vi "ep_Read Public Record Inf.vi"(8 "error in":errorcluster, 11 "task in":T2={"file refnums"=[], "Data Object"=refnum, "config info"={"station_name"="", "rec_dev_id"="", "rev_year"=1999.0, "TT"=0, "##A"=0, "##D"=0, "analog channel info"=[], "status channel info"=[], "lf"=50.0, "nrates"=0, "samp info"=[], "initial timestamp"=timestamp(0 s since 1904-01-01), "trigger timestamp"=timestamp(0 s since 1904-01-01), "ft"=enum."Binary", "timemult"=1.0}, "public inf content"={"Source"="", "Record Type"=enum."Unknown", "Phase ID"="", "Event Description"="", "Device ID"="", "Distance of Fault"=-1.0, "Distance Unit"=enum."Miles", "Max_Current"=inf, "Min_Current"=-inf, "Max_Voltage"=inf, "Min_Voltage"=-inf, "EventNoteCount"=0, "Event Information"=[]}, "private inf content"=[], "internal buffers"={"start index"=1, "config to public inf"=enum."disabled", "static config info"="", "static file_des record inf"="", "static file_des channel inf"="", "public inf"="", "private inf"=""}} {"public inf content"."Event Information"."min sample number" max=9999999999; "public inf content"."Event Information"."max sample number" max=9999999999; "config info"."nrates" max=999; "config info"."status channel info"."Dn" min=1 max=999999; "config info"."analog channel info"."An" min=1 max=999999; "config info"."trigger timestamp" format="%<%H:%M:%S%6u\n%d/%m/%Y>T"; "config info"."initial timestamp" format="%<%H:%M:%S%6u\n%d/%m/%Y>T"; "config info"."##D" max=999999; "config info"."##A" max=999999; "config info"."TT" min=1 max=999999; "config info"."rev_year" min=1999.0 max=1999.0}) -> (0 "error out":errorcluster, 2 "public record information":T1={"source"="", "record type"=enum."Unknown", "phase ID"="", "event description"="", "device ID"="", "distance of fault"=-1.0, "distance unit"=enum."Miles", "max current"=inf, "min current"=-inf, "max voltage"=inf, "min voltage"=-inf}, 3 "task out":T2={"file refnums"=[], "Data Object"=refnum, "config info"={"station_name"="", "rec_dev_id"="", "rev_year"=1999.0, "TT"=0, "##A"=0, "##D"=0, "analog channel info"=[], "status channel info"=[], "lf"=50.0, "nrates"=0, "samp info"=[], "initial timestamp"=timestamp(0 s since 1904-01-01), "trigger timestamp"=timestamp(0 s since 1904-01-01), "ft"=enum."Binary", "timemult"=1.0}, "public inf content"={"Source"="", "Record Type"=enum."Unknown", "Phase ID"="", "Event Description"="", "Device ID"="", "Distance of Fault"=-1.0, "Distance Unit"=enum."Miles", "Max_Current"=inf, "Min_Current"=-inf, "Max_Voltage"=inf, "Min_Voltage"=-inf, "EventNoteCount"=0, "Event Information"=[]}, "private inf content"=[], "internal buffers"={"start index"=1, "config to public inf"=enum."disabled", "static config info"="", "static file_des record inf"="", "static file_des channel inf"="", "public inf"="", "private inf"=""}} {"public inf content"."Event Information"."min sample number" max=9999999999; "public inf content"."Event Information"."max sample number" max=9999999999; "config info"."nrates" max=999; "config info"."status channel info"."Dn" min=1 max=999999; "config info"."analog channel info"."An" min=1 max=999999; "config info"."trigger timestamp" format="%<%H:%M:%S%6u\n%d/%m/%Y>T"; "config info"."initial timestamp" format="%<%H:%M:%S%6u\n%d/%m/%Y>T"; "config info"."##D" max=999999; "config info"."##A" max=999999; "config info"."TT" min=1 max=999999; "config info"."rev_year" min=1999.0 max=1999.0})   [LabVIEW 2011, in "NI_EP_COMTRADE.lvlib"]
uses:
  <vilib>/addons/Electrical Power/File IO/NI_EP_COMTRADE.lvlib
  <vilib>/addons/Electrical Power/File IO/COMTRADE/typedefs/ep_Task.ctl
  <vilib>/addons/Electrical Power/File IO/COMTRADE/typedefs/ep_Config Info.ctl
  <vilib>/addons/Electrical Power/File IO/COMTRADE/typedefs/ep_Analog Channel Info.ctl
  <vilib>/addons/Electrical Power/File IO/COMTRADE/typedefs/ep_Status Channel Info.ctl
  <vilib>/addons/Electrical Power/File IO/COMTRADE/typedefs/ep_File Format.ctl
  <vilib>/addons/Electrical Power/File IO/COMTRADE/typedefs/ep_Public Inf Content.ctl
  <vilib>/addons/Electrical Power/File IO/COMTRADE/typedefs/ep_Public Event Inf.ctl
  <vilib>/addons/Electrical Power/File IO/COMTRADE/typedefs/ep_Private Inf Content.ctl
  <vilib>/addons/Electrical Power/File IO/COMTRADE/typedefs/ep_Public Record Inf.ctl
  <vilib>/Platform/storage/Storage.llb/Get Property (Storage Refnums).vi
  <vilib>/Platform/storage/Storage.llb/Get Property (String).vi
  <vilib>/Platform/storage/Storage.llb/Get Property (DBL).vi
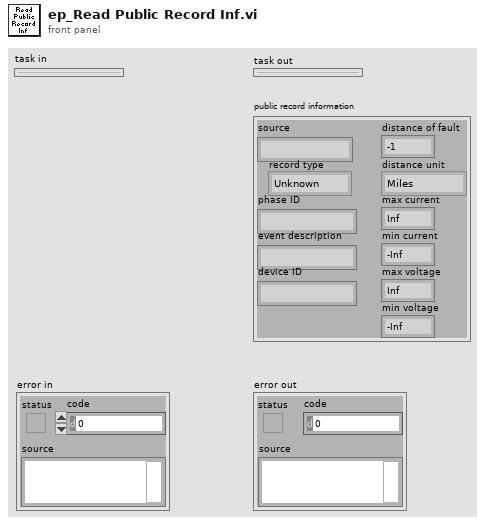
[diagram p1: front panel]
types:
  T1 = typedef "NI_EP_COMTRADE.lvlib/ep_Public Record Inf.ctl" = cluster{"source":string, "record type":enum16{"Fault", "Unknown", "Misoperation", "Close", "Trip", "Reclose", "Power swing", "Simulation"}, "phase ID":string, "event description":string, "device ID":string, "distance of fault":dbl, "distance unit":enum16{"Miles", "Kilometers", "Percent of line", "Percent of setting", "Ohms"}, "max current":dbl, "min current":dbl, "max voltage":dbl, "min voltage":dbl}
  T2 = typedef "NI_EP_COMTRADE.lvlib/ep_Task.ctl" = cluster{"file refnums":refnum<file>[], "Data Object":refnum<k20>, "config info":T3, "public inf content":T7, "private inf content":T9, "internal buffers":cluster{"start index":u32, "config to public inf":enum16{"disabled", "enabled", "buffered"}, "static config info":string, "static file_des record inf":string, "static file_des channel inf":string, "public inf":string, "private inf":string}}
  T3 = typedef "NI_EP_COMTRADE.lvlib/ep_Config Info.ctl" = cluster{"station_name":string, "rec_dev_id":string, "rev_year":dbl, "TT":u32, "##A":u32, "##D":u32, "analog channel info":T4[], "status channel info":T5[], "lf":sgl, "nrates":u16, "samp info":cluster{"samp":sgl, "endsamp":u32}[], "initial timestamp":timestamp, "trigger timestamp":timestamp, "ft":T6, "timemult":sgl}
  T4 = typedef "NI_EP_COMTRADE.lvlib/ep_Analog Channel Info.ctl" = cluster{"An":u32, "ch_id":string, "ph":string, "ccbm":string, "uu":string, "a":sgl, "b":sgl, "skew":sgl, "min":i32, "max":i32, "primary":sgl, "secondary":sgl, "PS":enum16{"P", "S"}}
  T5 = typedef "NI_EP_COMTRADE.lvlib/ep_Status Channel Info.ctl" = cluster{"Dn":u32, "ch_id":string, "ph":string, "ccbm":string, "Y":bool}
  T6 = typedef "NI_EP_COMTRADE.lvlib/ep_File Format.ctl" = enum16{"ASCII", "Binary"}
  T7 = typedef "NI_EP_COMTRADE.lvlib/ep_Public Inf Content.ctl" = cluster{"Source":string, "Record Type":enum16{"Fault", "Unknown", "Misoperation", "Close", "Trip", "Reclose", "Power swing", "Simulation"}, "Phase ID":string, "Event Description":string, "Device ID":string, "Distance of Fault":dbl, "Distance Unit":enum16{"Miles", "Kilometers", "Percent of line", "Percent of setting", "Ohms"}, "Max_Current":dbl, "Min_Current":dbl, "Max_Voltage":dbl, "Min_Voltage":dbl, "EventNoteCount":u32, "Event Information":T8[]}
  T8 = typedef "NI_EP_COMTRADE.lvlib/ep_Public Event Inf.ctl" = cluster{"channel number":u32, "max value":dbl, "min value":dbl, "max sample number":u64, "min sample number":u64, "max sample text":string[], "min sample text":string[]}
  T9 = typedef "NI_EP_COMTRADE.lvlib/ep_Private Inf Content.ctl" = cluster{"Section Header":string, "Entry Names":string[], "Entry Values":string[]}[]
  T10 = enum16{"Miles", "Kilometers", "Percent of line", "Percent of setting", "Ohms"}
  T11 = enum16{"Fault", "Unknown", "Misoperation", "Close", "Trip", "Reclose", "Power swing", "Simulation"}
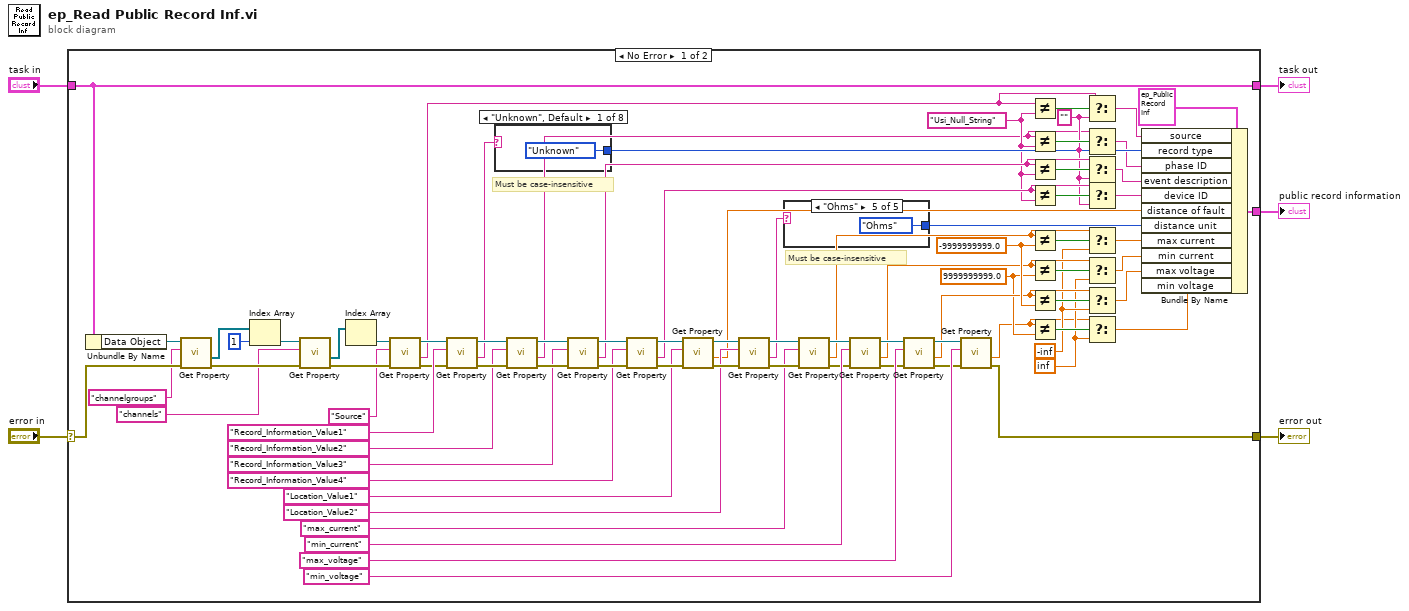
[diagram p0: block diagram]
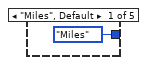
[diagram p2: hidden frame]
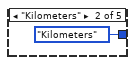
[diagram p3: hidden frame]
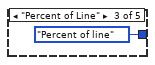
[diagram p4: hidden frame]
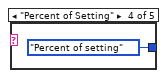
[diagram p5: hidden frame]
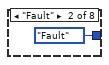
[diagram p6: hidden frame]
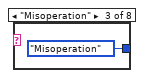
[diagram p7: hidden frame]
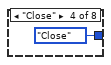
[diagram p8: hidden frame]
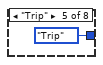
[diagram p9: hidden frame]
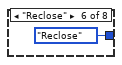
[diagram p10: hidden frame]
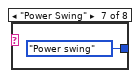
[diagram p11: hidden frame]
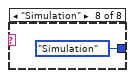
[diagram p12: hidden frame]
diagram:
  n1 = case shown="No Error" "error in" {
    selector: "error in" -> [w81 w100]
    tunnel: "task in" -> [w86 w101]
    tunnel: [w86 w101] -> w3
    tunnel: [w75 w100] -> w2
    tunnel: [w83 _] -> w1
    frame No Error {
      w10 = "" ("f")
      w9 = "Usi_Null_String" ("x")
      w28 = -9999999999.0
      w24 = 9999999999.0
      w23 = -inf
      w22 = inf
      # "Must be case-insensitive"
      # "Must be case-insensitive"
      n2 = Unbundle By Name(w86) -> ("Data Object"=w82:refnum<k20>)
      n3 = call-poly <vilib>:"Get Property.vi"("error in (no error)"=w81, "Property name"="channelgroups", "storage refnum"=w82) -> ("error out"=w79:errorcluster, "Value"=w85:refnum<k20>[])  [unwired: 6 in, 1 out]
      n4 = Index Array(array=w85, index=1) -> (element=w80:refnum<k20>)
      n5 = call-poly <vilib>:"Get Property.vi"("error in (no error)"=w79, "Property name"="channels", "storage refnum"=w80) -> ("error out"=w78:errorcluster, "Value"=w74:refnum<k20>[])  [unwired: 6 in, 1 out]
      n6 = Index Array(array=w74) -> (element=w44:refnum<k20>)  [unwired: 1 in]
      n7 = call-poly <vilib>:"Get Property.vi"("error in (no error)"=w78, "Property name"="Source", "storage refnum"=w44) -> ("error out"=w42:errorcluster, "Value"=w7:string, "storage refnum out"=w43:refnum<k20>)  [unwired: 6 in]
      n8 = call-poly <vilib>:"Get Property.vi"("error in (no error)"=w42, "Property name"="Record_Information_Value1", "storage refnum"=w43) -> ("error out"=w65:errorcluster, "Value"=w49:string, "storage refnum out"=w66:refnum<k20>)  [unwired: 6 in]
      n9 = case shown="\"Unknown\", Default" w49 {
        tunnel: [T11."Unknown" ("Record Type") T11."Fault" ("Record Type") T11."Misoperation" ("Record Type") T11."Close" ("Record Type") T11."Trip" ("Record Type") T11."Reclose" ("Record Type") T11."Power swing" ("Record Type") T11."Simulation" ("Record Type")] -> w47
        frame "Unknown", Default {
        }
        frame "Fault" {
        }
        frame "Misoperation" {
        }
        frame "Close" {
        }
        frame "Trip" {
        }
        frame "Reclose" {
        }
        frame "Power Swing" {
        }
        frame "Simulation" {
        }
      }
      n10 = call-poly <vilib>:"Get Property.vi"("error in (no error)"=w65, "Property name"="Record_Information_Value2", "storage refnum"=w66) -> ("error out"=w70:errorcluster, "Value"=w8:string, "storage refnum out"=w69:refnum<k20>)  [unwired: 6 in]
      n11 = call-poly <vilib>:"Get Property.vi"("error in (no error)"=w70, "Property name"="Record_Information_Value3", "storage refnum"=w69) -> ("error out"=w68:errorcluster, "Value"=w11:string, "storage refnum out"=w67:refnum<k20>)  [unwired: 6 in]
      n12 = call-poly <vilib>:"Get Property.vi"("error in (no error)"=w68, "Property name"="Record_Information_Value4", "storage refnum"=w67) -> ("error out"=w61:errorcluster, "Value"=w12:string, "storage refnum out"=w60:refnum<k20>)  [unwired: 6 in]
      n13 = call-poly <vilib>:"Get Property.vi"("error in (no error)"=w61, "Property name"="Location_Value1", "storage refnum"=w60) -> ("error out"=w57:errorcluster, "Value"=w48:dbl, "storage refnum out"=w58:refnum<k20>)  [unwired: 6 in]
      n14 = call-poly <vilib>:"Get Property.vi"("error in (no error)"=w57, "Property name"="Location_Value2", "storage refnum"=w58) -> ("error out"=w56:errorcluster, "Value"=w46:string, "storage refnum out"=w55:refnum<k20>)  [unwired: 6 in]
      n15 = case shown="\"Ohms\"" w46 {
        tunnel: [T10."Miles" ("Distance Unit") T10."Kilometers" ("Distance Unit") T10."Percent of line" ("Distance Unit") T10."Percent of setting" ("Distance Unit") T10."Ohms" ("Distance Unit")] -> w45
        frame "Miles", Default {
        }
        frame "Kilometers" {
        }
        frame "Percent of Line" {
        }
        frame "Percent of Setting" {
        }
        frame "Ohms" {
        }
      }
      n16 = call-poly <vilib>:"Get Property.vi"("error in (no error)"=w56, "Property name"="max_current", "storage refnum"=w55) -> ("error out"=w35:errorcluster, "Value"=w27:dbl, "storage refnum out"=w37:refnum<k20>)  [unwired: 6 in]
      n17 = call-poly <vilib>:"Get Property.vi"("error in (no error)"=w35, "Property name"="min_current", "storage refnum"=w37) -> ("error out"=w30:errorcluster, "Value"=w26:dbl, "storage refnum out"=w36:refnum<k20>)  [unwired: 6 in]
      n18 = call-poly <vilib>:"Get Property.vi"("error in (no error)"=w30, "Property name"="max_voltage", "storage refnum"=w36) -> ("error out"=w29:errorcluster, "Value"=w25:dbl, "storage refnum out"=w38:refnum<k20>)  [unwired: 6 in]
      n19 = call-poly <vilib>:"Get Property.vi"("error in (no error)"=w29, "Property name"="min_voltage", "storage refnum"=w38) -> ("error out"=w75:errorcluster, "Value"=w21:dbl)  [unwired: 6 in, 1 out]
      n20 = Not Equal?(x=w7, y=w9) -> (x != y?=w20:bool)
      n21 = Not Equal?(x=w8, y=w9) -> (x != y?=w18:bool)
      n22 = Not Equal?(x=w11, y=w9) -> (x != y?=w17:bool)
      n23 = Not Equal?(x=w12, y=w9) -> (x != y?=w15:bool)
      n24 = Not Equal?(x=w27, y=w28) -> (x != y?=w34:bool)
      n25 = Not Equal?(x=w26, y=w24) -> (x != y?=w33:bool)
      n26 = Not Equal?(x=w25, y=w28) -> (x != y?=w32:bool)
      n27 = Not Equal?(x=w21, y=w24) -> (x != y?=w31:bool)
      n28 = Select(t=w7, s=w20, f=w10) -> (s? t:f=w19:string)
      n29 = Select(t=w8, s=w18, f=w10) -> (s? t:f=w6:string)
      n30 = Select(t=w11, s=w17, f=w10) -> (s? t:f=w16:string)
      n31 = Select(t=w12, s=w15, f=w10) -> (s? t:f=w13:string)
      n32 = Select(t=w27, s=w34, f=w23) -> (s? t:f=w14:dbl)
      n33 = Select(t=w26, s=w33, f=w22) -> (s? t:f=w41:dbl)
      n34 = Select(t=w25, s=w32, f=w23) -> (s? t:f=w40:dbl)
      n35 = Select(t=w21, s=w31, f=w22) -> (s? t:f=w39:dbl)
      n36 = Bundle By Name(cluster=T1 {"source"="", "record type"=enum."Unknown", "phase ID"="", "event description"="", "device ID"="", "distance of fault"=-1.0, "distance unit"=enum."Miles", "max current"=-inf, "min current"=inf, "max voltage"=-inf, "min voltage"=inf} ("public record information"), "source"=w19, "record type"=w47, "phase ID"=w6, "event description"=w16, "device ID"=w13, "distance of fault"=w48, "distance unit"=w45, "max current"=w14, "min current"=w41, "max voltage"=w40, "min voltage"=w39) -> (w83:T1)
    }
    frame Error {
    }
  }
  "task out" <- w3
  "error out" <- w2
  "public record information" <- w1
